vi "attribute_read.vi"(5 "Repeated Capability":string, 7 "Attribute ID":string, 8 "error in":errorcluster, 11 "VISA resource name":refnum<visa-resource-name>) -> (0 "error out":errorcluster, 1 "Double out":dbl, 2 "I32 out":i32, 3 "VISA resource name out":refnum<visa-resource-name>, 4 "Boolean out":bool, 6 "String out":string, 9 "I64 out":i64)   [LabVIEW 2014, in "rszvl_rsidr_core.lvlib"]
uses:
  rszvl_rsidr_core.lvlib
  type_Error_Codes.ctl
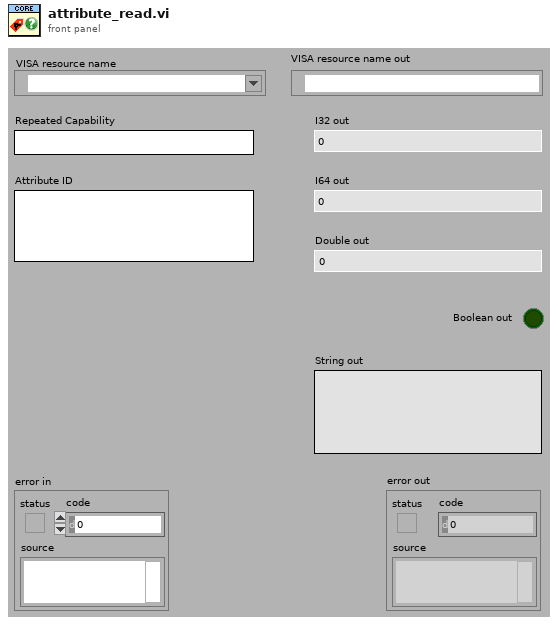
[diagram p1: front panel]
types:
  T1 = typedef "rszvl_rsidr_core.lvlib/type_Error_Codes.ctl" = enum16{"No_error", "VISA_err_ResourceNotFound", "VISA_err_Timeout", "VISA_warn_MoreDataAvailable", "RS_err_MissingCallback", "RS_err_InvalidAttribute", "RS_err_InvalidValue", "RS_err_UnknownResource", "RS_err_AlreadyInitialized", "RS_err_InstrumentStatus", "RS_err_BadRepCapName", "RS_err_TypesMismatch", "RS_err_ValueNotSupported", "RS_err_InvalidRngTable", "RS_err_IDqueryFail", "RS_err_UnexpResponse", "VISA_warn_ConfigNotLoaded", "RS_err_AttributeNotReadable", "RS_err_AttributeNotWritable", "RS_err_InstrumentType", "RS_err_InstrumentOption", "VISA_err_InvalidSize", "RS_err_ReliabilityIndicator", "VISA_warn_UnknownStatus", "VISA_warn_TermCharRead", "VISA_err_IO_error"}
  T2 = typedef "rszvl_rsidr_core.lvlib/type_Attribute.ctl" = cluster{"Identifier":string, "Descriptive name":string, "Data Type":T3, "Command":string, "Access":u16, "Range Table":string, "Read Callback":string, "Write Callback":string, "Range Callback":string, "Check Callback":string, "Rngtable Callback":string, "Coerce Callback":string, "Supported Models":string, "Instrument Options":string, "Repeated Capabilities":string, "Check Status Callback":string, "Index":i32, "Flag: OPC Wait":bool, "Flag: Dont check status":bool, "Flag: Cache Only":bool}
  T3 = typedef "rszvl_rsidr_core.lvlib/type_Attribute_Data_Type.ctl" = enum16{"Integer 32", "Double", "String", "Boolean", "None", "Integer 64"}
  T4 = typedef "rszvl_rsidr_core.lvlib/type_Session_Data.ctl" = cluster{"Instr type":string, "Instr type for err. msg.":string, "Installed Options":string[], "OPC Timeout":i32, "Query Instrument Status":bool, "Check Range":bool, "Check Options":bool, "Add LF to Write":bool, "Simulate":bool, "Logging":bool, "Logging params":variant, "Interface Type":enum16{"Unknown", "GPIB", "VXI", "GPIB_VXI", "ASRL", "PXI", "TCPIP", "USB", "SOCKET"}, "Fast Sweep":i32, "AdditionalFlags":i32, "WaitBeforeWrite":i32, "WaitBeforeRead":i32, "BinDataChunkSize":i64}
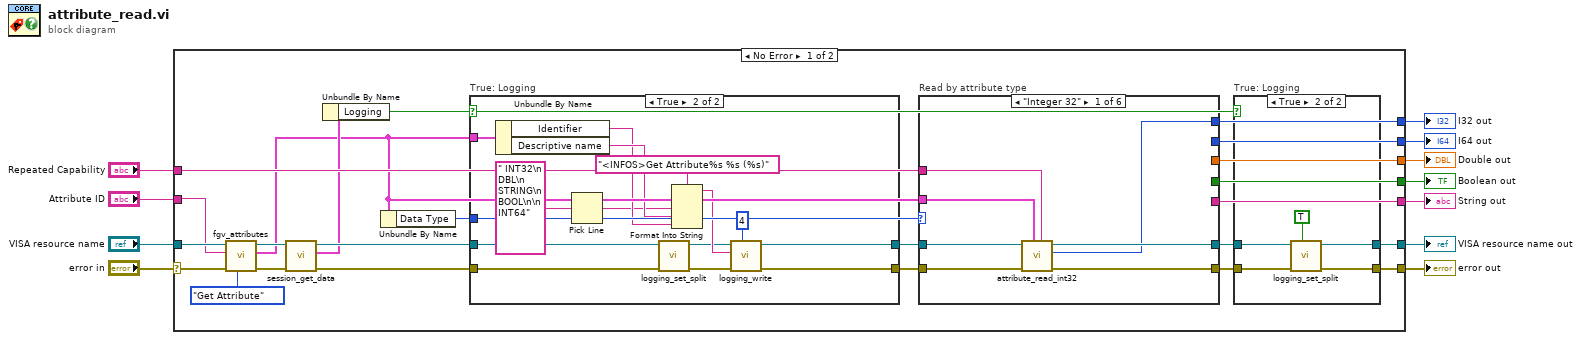
[diagram p0: block diagram]
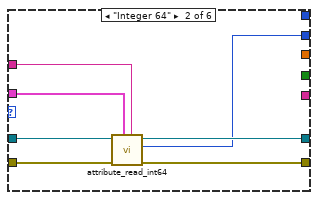
[diagram p4: hidden frame]
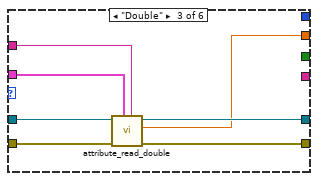
[diagram p5: hidden frame]
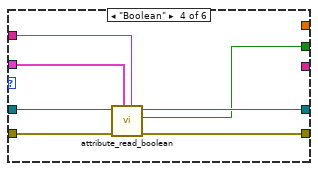
[diagram p6: hidden frame]
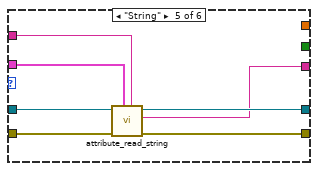
[diagram p7: hidden frame]
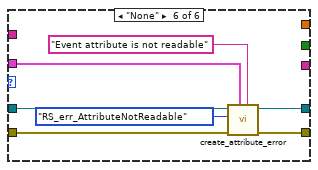
[diagram p8: hidden frame]
diagram:
  n1 = case shown="No Error" "error in" {
    selector: "error in" -> [w16 w101]
    tunnel: "VISA resource name" -> [w23 w102]
    tunnel: "Repeated Capability" -> [w34 _]
    tunnel: [w24 w102] -> w9
    tunnel: [w25 w101] -> w8
    tunnel: "Attribute ID" -> [w14 _]
    tunnel: [w33 _] -> w5
    tunnel: [w32 _] -> w4
    tunnel: [w31 _] -> w3
    tunnel: [w30 _] -> w2
    tunnel: [w29 _] -> w1
    frame No Error {
      n2 = call "fgv_attributes.vi"("Operation"=enum16{"Initialize", "Get Attribute"}."Get Attribute", "error in"=w16, "Attribute ID in"=w14) -> ("error out"=w15:errorcluster, "Attribute out"=w13:T2)  [unwired: 6 in, 1 out]
      n3 = call "session_get_data.vi"("error in"=w15, "VISA resource name"=w23) -> ("error out"=w22:errorcluster, "Session User Data out"=w18:T4, "VISA resource name out"=w21:refnum<visa-resource-name>)  [unwired: 7 in]
      n4 = Unbundle By Name(w18) -> ("Logging"=w20:bool)
      n5 = Unbundle By Name(w13) -> ("Data Type"=w19:T3)
      n6 = case "True: Logging" shown="True" w20 {
        tunnel: w22 -> [w35 w39]
        tunnel: w13 -> [_ w51]
        tunnel: w21 -> [w36 w40]
        tunnel: [w36 w42] -> w28
        tunnel: w19 -> [_ w46]
        tunnel: [w35 w41] -> w17
        frame False {
        }
        frame True {
          n7 = Unbundle By Name(w51) -> ("Identifier"=w48:string, "Descriptive name"=w49:string)
          n8 = Pick Line(multi-line string=" INT32\n DBL\n STRING\n BOOL\n\n INT64", line index=w46) -> (output string=w45:string)  [unwired: 1 in]
          n9 = call "logging_set_split.vi"("error in"=w39, "VISA resource name"=w40) -> ("error out"=w38:errorcluster, "VISA resource name out"=w37:refnum<visa-resource-name>)  [unwired: 8 in]
          n10 = Format Into String(format string="<INFOS>Get Attribute%s %s (%s)", w45, w49, w48) -> (resulting string=w47:string)  [unwired: 2 in, 1 out]
          n11 = call "logging_write.vi"("Add call chain offset\n(No call chain)"=4 ("Add call chain offset\n(No call chain)"), "error in"=w38, "String to write"=w47, "VISA resource name"=w37) -> ("error out"=w41:errorcluster, "VISA resource name out"=w42:refnum<visa-resource-name>)  [unwired: 6 in]
        }
      }
      n12 = case "Read by attribute type" shown="\"Integer 32\"" w19 {
        tunnel: w13 -> [w59 w67 w73 w81 w88 w98]
        tunnel: w28 -> [w65 w72 w79 w86 w93 w97]
        tunnel: w17 -> [w64 w71 w78 w85 w92 w100]
        tunnel: w34 -> [w60 w68 w74 w82 w89 _]
        tunnel: [w63 w70 w77 w84 w91 w96] -> w26
        tunnel: [w62 w69 w76 w83 w90 w99] -> w27
        tunnel: [w61 _ _ _ _ _] -> w33
        tunnel: [_ w66 _ _ _ _] -> w32
        tunnel: [_ _ w75 _ _ _] -> w31
        tunnel: [_ _ _ w80 _ _] -> w30
        tunnel: [_ _ _ _ w87 _] -> w29
        frame "Integer 32" {
          n13 = call "attribute_read_int32.vi"("Repeated Capability"=w60, "Attribute"=w59, "error in"=w64, "VISA resource name"=w65) -> ("error out"=w62:errorcluster, "I32 out"=w61:i32, "VISA resource name out"=w63:refnum<visa-resource-name>)  [unwired: 5 in]
        }
        frame "Integer 64" {
          n14 = call "attribute_read_int64.vi"("Repeated Capability"=w68, "Attribute"=w67, "error in"=w71, "VISA resource name"=w72) -> ("error out"=w69:errorcluster, "int64 out"=w66:i64, "VISA resource name out"=w70:refnum<visa-resource-name>)  [unwired: 5 in]
        }
        frame "Double" {
          n15 = call "attribute_read_double.vi"("Repeated Capability"=w74, "Attribute"=w73, "error in"=w78, "VISA resource name"=w79) -> ("error out"=w76:errorcluster, "double out"=w75:dbl, "VISA resource name out"=w77:refnum<visa-resource-name>)  [unwired: 5 in]
        }
        frame "Boolean" {
          n16 = call "attribute_read_boolean.vi"("Repeated Capability"=w82, "Attribute"=w81, "error in"=w85, "VISA resource name"=w86) -> ("error out"=w83:errorcluster, "boolean out"=w80:bool, "VISA resource name out"=w84:refnum<visa-resource-name>)  [unwired: 5 in]
        }
        frame "String" {
          n17 = call "attribute_read_string.vi"("Repeated Capability"=w89, "Attribute"=w88, "error in"=w92, "VISA resource name"=w93) -> ("error out"=w90:errorcluster, "string out"=w87:string, "VISA resource name out"=w91:refnum<visa-resource-name>)  [unwired: 5 in]
        }
        frame "None" {
          n18 = call "create_attribute_error.vi"("Error Elaboration (\"\")"="Event attribute is not readable" ("Error Elaboration"), "Attribute"=w98, "error in"=w100, "Error Enum in"=type_Error_Codes."RS_err_AttributeNotReadable" ("Error Enum in (from err to recompose)"), "VISA resource name"=w97) -> ("error out"=w99:errorcluster, "VISA resource name out"=w96:refnum<visa-resource-name>)  [unwired: 5 in]
        }
      }
      n19 = case "True: Logging" shown="True" w20 {
        tunnel: w27 -> [w53 w58]
        tunnel: [w53 w56] -> w25
        tunnel: w26 -> [w52 w57]
        tunnel: [w52 w55] -> w24
        frame False {
        }
        frame True {
          n20 = call "logging_set_split.vi"("Evaluate section error (F)"=TRUE, "error in"=w58, "VISA resource name"=w57) -> ("error out"=w56:errorcluster, "VISA resource name out"=w55:refnum<visa-resource-name>)  [unwired: 7 in]
        }
      }
    }
    frame Error {
    }
  }
  "error out" <- w8
  "VISA resource name out" <- w9
  "I64 out" <- w4
  "I32 out" <- w5
  "Double out" <- w3
  "String out" <- w1
  "Boolean out" <- w2
